vi "Set Connection Reference.vi"(8 "error in (no error)":errorcluster, 10 "TCP Network Connection":refnum<k5>, 11 "IP Connection in":refnum<class "IP Connection.lvclass">) -> (0 "error out":errorcluster, 3 "IP Connection out":refnum<class "IP Connection.lvclass">)   [LabVIEW 2011, in "Tinkerforge.lvlib" / "IP Connection.lvclass"]
doc: "This VI sets the connection reference of the IP Connection."
uses:
  IP Connection.lvclass
  IP Connection.lvclass/IP Connection.ctl
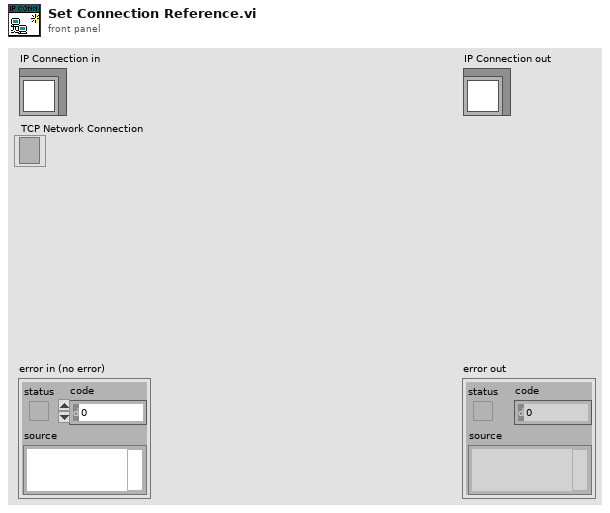
[diagram p1: front panel]
types:
  T1 = typedef "Tinkerforge.lvlib/IP Connection.lvclass/Connection.ctl" = cluster{"TCP Network Connection":refnum<k5>, "is connected":bool, "Connection Status":T2}
  T2 = typedef "Tinkerforge.lvlib/IP Connection.lvclass/Connection Status.ctl" = enum16{"Uninitialized", "Connected", "Reconnecting", "Disconnected"}
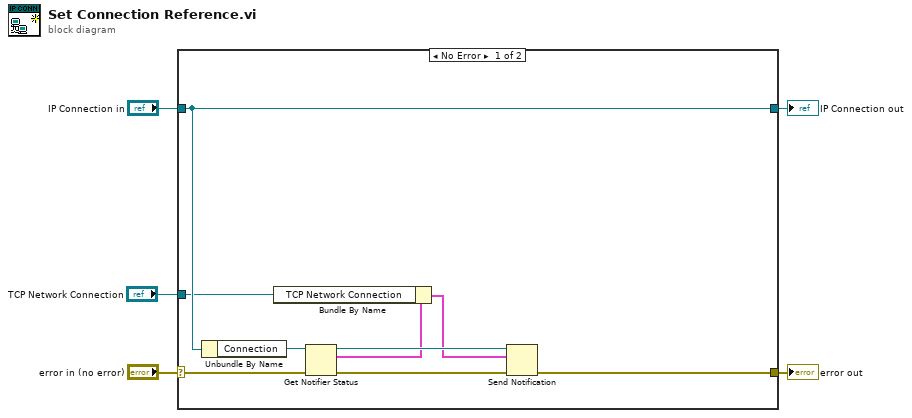
[diagram p0: block diagram]
diagram:
  n1 = case shown="No Error" "error in (no error)" {
    selector: "error in (no error)" -> [w10 w16]
    tunnel: [w12 w16] -> w4
    tunnel: [w14 w15] -> w2
    tunnel: "IP Connection in" -> [w14 w15]
    tunnel: "TCP Network Connection" -> [w6 _]
    frame No Error {
      n2 = Unbundle By Name(w14) -> ("Connection"=w13:refnum<notifier>)
      n3 = Get Notifier Status(notifier=w13, error in (no error)=w10) -> (notifier out=w11:refnum<notifier>, current notification=w8:T1, error out=w9:errorcluster)  [unwired: 2 out]
      n4 = Bundle By Name(cluster=w8, "TCP Network Connection"=w6) -> (w7:T1)
      n5 = Send Notification(notification=w7, notifier=w11, error in (no error)=w9) -> (error out=w12:errorcluster)  [unwired: 1 out]
    }
    frame Error {
    }
  }
  "error out" <- w4
  "IP Connection out" <- w2
